vi "to string.vi"(8 "error in":errorcluster, 11 "OPC UA configuration in":refnum<class "OPC UA Client configuration.lvclass">) -> (0 "error out":errorcluster, 1 "data":string, 2 "version":string, 3 "OPC UA configuration out":refnum<class "OPC UA Client configuration.lvclass">)   [LabVIEW 2013, in "OPC UA Client configuration.lvclass"]
doc: "Provides an interface for saving a module configuration to a file or other serialized data source. It is recommended that all children of this class store data in two sets--data required for its own initialization, and any data required for parent initialization--and that each implementation uses the <b>Call Parent Method</b> primitive to serialize parent information."
uses:
  OPC UA Client configuration.lvclass
  <vilib>/NI/Tag Bus Module Framework/module configuration/TBM module configuration.lvclass
  OPC UA Client configuration.lvclass/OPC UA Client configuration.ctl
  current version.vi
  <vilib>/NI/Configuration Framework/serializable configuration/NISE_CEF_serializable configuration.lvclass
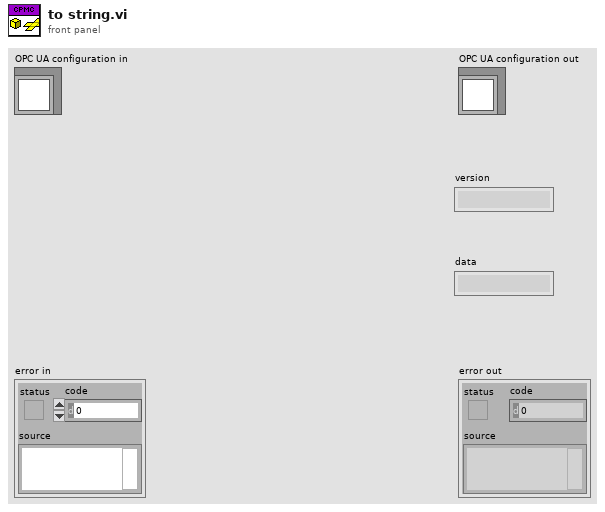
[diagram p1: front panel]
types:
  T1 = typedef "OPC UA Client configuration.lvclass/OPC UA Data Type.ctl" = u16
  T2 = cluster{"channel":refnum<class "TBM channel.lvclass">, "Node Path":string, "OPC UA Data Type":T1}[]
  T3 = typedef "OPC UA Client configuration.lvclass/Client Connection Configuration.ctl" = cluster{"Server Certificates":cluster{"Relative Path?":bool, "Certificate Paths":path[], "Certificate Names":string[]}, "Client Certificates":cluster{"Relative Path?":bool, "Certificate Paths":path[], "Certificate Names":string[]}, "Client Configuration":cluster{"Server Endpoint URL":string, "Security Policy":cluster{"Message Mode":enum16{"None", "Sign", "Sign and Encrypt"}, "Security":enum16{"Basic256", "Basic128Rsa15"}}, "Username/Password":cluster{"Username":string, "Password":string}}}
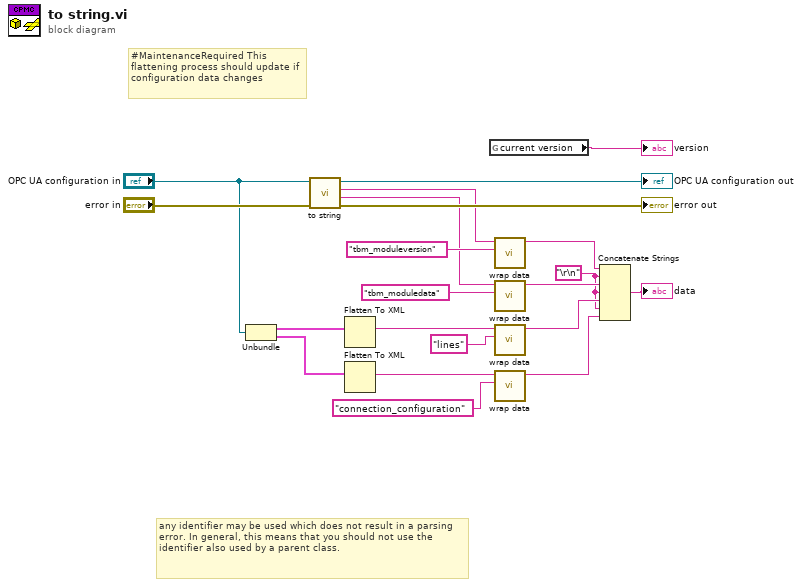
[diagram p0: block diagram]
diagram:
  w2 = "\r\n"
  # "any identifier may be used which does not result in a parsing error. In general, this means that you should not use the identifier also used by a parent class."
  # "#MaintenanceRequired This flattening process should update if configuration data changes"
  n1 = Unbundle("OPC UA configuration in") -> (w7:T2, w5:T3)
  n2 = call-parent "to string.vi"("error in"="error in", "module configuration in"="OPC UA configuration in") -> ("error out"=→"error out":errorcluster, "data"=w12:string, "version"=w13:string, "module configuration out"=→"OPC UA configuration out":refnum<class "OPC UA Client configuration.lvclass">)  [unwired: 6 in]
  n3 = Flatten To XML(anything=w7) -> (xml string=w6:string)
  n4 = Flatten To XML(anything=w5) -> (xml string=w4:string)
  n5 = global read "current version.vi" "current version"() -> (→"version":string)
  n6 = call <vilib>:"wrap data.vi"("identifier"="tbm_moduleversion" ("additional identifier"), "data to wrap"=w13) -> ("wrapped data"=w15:string)  [unwired: 9 in]
  n7 = call <vilib>:"wrap data.vi"("identifier"="tbm_moduledata" ("additional identifier"), "data to wrap"=w12) -> ("wrapped data"=w14:string)  [unwired: 9 in]
  n8 = call <vilib>:"wrap data.vi"("identifier"="lines" ("additional identifier"), "data to wrap"=w6) -> ("wrapped data"=w9:string)  [unwired: 9 in]
  n9 = call <vilib>:"wrap data.vi"("identifier"="connection_configuration" ("additional identifier"), "data to wrap"=w4) -> ("wrapped data"=w1:string)  [unwired: 9 in]
  n10 = Concatenate Strings(w15, w2, w14, w2, w9, w2, w1) -> (→"data":string)
